vi "archive log.vi"(4 "error in (no error)":errorcluster, 6 "Flat Log (\"\")":string, 7 "Log Path (empty)":path) -> (0 "error out":errorcluster)   [LabVIEW 2011]
uses:
  Summitek EXT/OpenG EXT/file/file.llb/Strip Path Extension - String__ogtk.vi
  Summitek EXT/OpenG EXT/file/file.llb/File Exists - Scalar__ogtk.vi
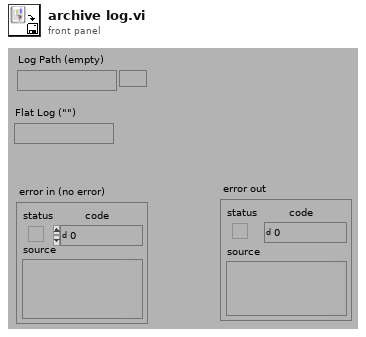
[diagram p1: front panel]
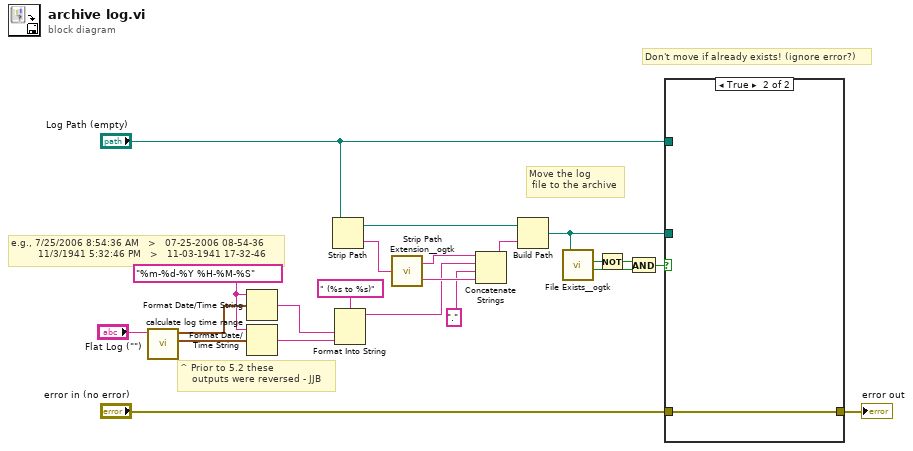
[diagram p0: block diagram]
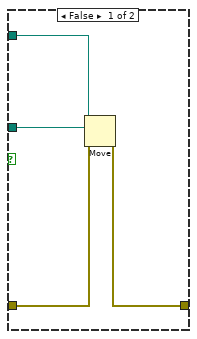
[diagram p2: hidden frame]
diagram:
  w1 = "%m-%d-%Y %H-%M-%S" ("time format string (%c)")
  # "^ Prior to 5.2 these\n    outputs were reversed - JJB"
  # "e.g., 7/25/2006 8:54:36 AM   >   07-25-2006 08-54-36\n         11/3/1941 5:32:46 PM   >   11-03-1941 17-32-46"
  # "Don't move if already exists! (ignore error?)"
  # "Move the log\n file to the archive"
  n1 = call "calculate log time range.vi"("Log Contents (\"\")"="Flat Log (\"\")") -> ("Log Stop Time"=w2:timestamp, "Log Start Time"=w5:timestamp)  [unwired: 5 out]
  n2 = Format Date/Time String(time format string (%c)=w1, seconds (now)=w5) -> (date/time string=w3:string)  [unwired: 1 in]
  n3 = Format Date/Time String(time format string (%c)=w1, seconds (now)=w2) -> (date/time string=w4:string)  [unwired: 1 in]
  n4 = Strip Path(path="Log Path (empty)") -> (stripped path=w18:path, name=w19:string)
  n5 = Format Into String(format string=" (%s to %s)", w3, w4) -> (resulting string=w16:string)  [unwired: 2 in, 1 out]
  n6 = call-poly "Strip Path Extension__ogtk.vi"("path"=w19) -> ("root"=w22:string, "extension"=w21:string)
  n7 = Concatenate Strings(w22, w16, ".", w21) -> (w20:string)
  n8 = Build Path(base path=w18, name or relative path=w20) -> (appended path=w13:path)
  n9 = call-poly "File Exists__ogtk.vi"("file path"=w13) -> ("is directory"=w12:bool, "exists"=w11:bool)  [unwired: 6 in]
  n10 = Not(x=w12) -> (.not. x?=w10:bool)
  n11 = And(x=w10, y=w11) -> (x .and. y?=w7:bool)
  n12 = case shown="True" w7 {
    tunnel: "Log Path (empty)" -> [w26 _]
    tunnel: w13 -> [w25 _]
    tunnel: "error in (no error)" -> [w24 w27]
    tunnel: [w23 w27] -> w8
    frame False {
      n13 = Move(source path=w26, error in=w24, 10:w25) -> (error out=w23:errorcluster)  [unwired: 4 out]
    }
    frame True {
    }
  }
  "error out" <- w8
